vi "STM Read Message (UDP).vi"(6 "Options":T1={"Ignore Timeout Error"=TRUE, "timeout ms (1000)"=1000, "max size (548)"=548}, 8 "error in":errorcluster, 11 "Connection Info":T3) -> (0 "error out":errorcluster, 1 "Name":T4, 2 "data string":string, 3 "Connection Info Out":T3, 4 "Data Info":T2, 5 "Timed Out?":bool)   [LabVIEW 2010]
doc: "This VI reads an incoming package of data from a host. This VI parses the package and extracts the data name and type as described in the meta data.\n\nFor the package to be parsed correctly, the meta data must be consistent in both the sender and the receiver. The data is packaged based on the existing meta data on the sender. \n\nUse the \"STM Read Meta Data\" and \"STM Write Meta Data\" VIs to ensure that both client and server have the same meta data.\n\nThe data is returned as a string. It is the responsibility of the user to cast it to the appropriate type.\n\nCopyright 2015, 2016, 2017 National Instruments Corporation\n\nLicensed under the Apache License, Version 2.0 (the \"License\"); you may not use this file except in compliance with the License.\n\n You may obtain a copy of the License at\n\n http://www.apache.org/licenses/LICENSE-2.0\n\nUnless required by applicable law or agreed to in writing, software distributed under the License is distributed on an \"AS IS\" BASIS, WITHOUT WARRANTIES OR CONDITIONS OF ANY KIND, either express or implied.\n\nSee the License for the specific language governing permissions and limitations under the License."
uses:
  stm_MetaDataElement.ctl
  stm_UDP Connection Info.ctl
  stm_UDP Data Info.ctl
  stm_UDP Read Options.ctl
  NI STM.lvlib
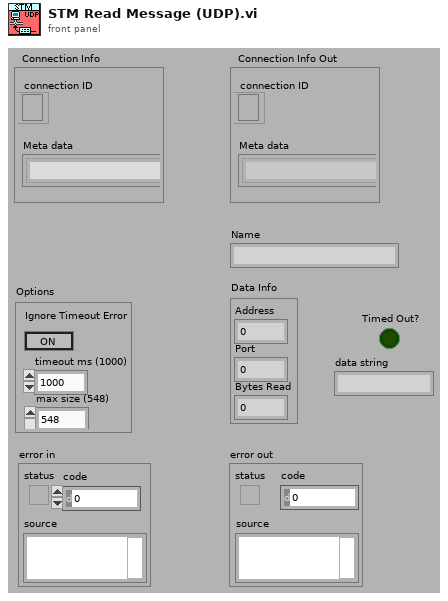
[diagram p1: front panel]
types:
  T1 = typedef "stm_UDP Read Options.ctl" = cluster{"Ignore Timeout Error":bool, "timeout ms (1000)":i32, "max size (548)":i32}
  T2 = typedef "stm_UDP Data Info.ctl" = cluster{"Address":u32, "Port":u16, "Bytes Read":i32}
  T3 = typedef "stm_UDP Connection Info.ctl" = cluster{"connection ID":refnum<k16>, "Meta data":T4[]}
  T4 = typedef "stm_MetaDataElement.ctl" = string
  T5 = typedef "NI STM.lvlib/MetaDataElement.ctl" = string
  T6 = typedef "NI STM.lvlib/UDP Connection Info.ctl" = cluster{"connection ID":refnum<k16>, "meta data":T5[]}
  T7 = typedef "NI STM.lvlib/UDP Data Info.ctl" = cluster{"address":u32, "port":u16, "bytes read":i32}
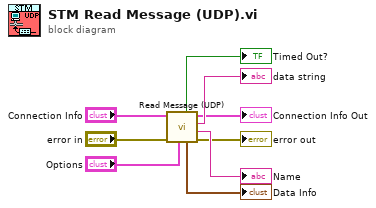
[diagram p0: block diagram]
diagram:
  n1 = call "Read Message (UDP).vi"("options"="Options", "error in"="error in", "connection info in"="Connection Info") -> ("error out"=→"error out":errorcluster, "name"=→"Name":T5, "data string"=→"data string":string, "connection info out"=→"Connection Info Out":T6, "data info"=→"Data Info":T7, "timed out?"=→"Timed Out?":bool)  [unwired: 3 in]
